vi "时间节点解密.vi"(10 "已延期":bool, 11 "输入密码":string) -> ()   [LabVIEW 2013]
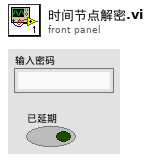
[diagram p1: front panel]
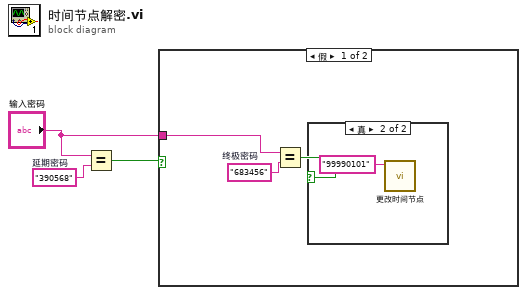
[diagram p0: block diagram]
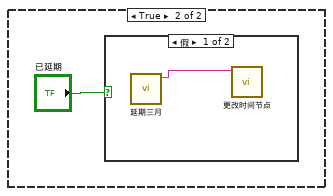
[diagram p3: hidden frame]
diagram:
  w3 = "390568"  # 延期密码
  n1 = Equal?(x="输入密码", y=w3) -> (x = y?=w2:bool)
  n2 = case shown="假" w2 {
    tunnel: "输入密码" -> [w5 _]
    frame False {
      w6 = "683456"  # 终极密码
      n3 = Equal?(x=w5, y=w6) -> (x = y?=w4:bool)
      n4 = case shown="真" w4 {
        frame False {
        }
        frame True {
          n5 = call "更改时间节点.vi"("时间字符串"="99990101") -> ()  [unwired: 10 in, 1 out]
        }
      }
    }
    frame True {
      n6 = case shown="假" "已延期" {
        frame False {
          n7 = call "延期三月.vi"() -> ("十进制整型字符串"=w9:string)  [unwired: 11 in]
          n8 = call "更改时间节点.vi"("时间字符串"=w9) -> ()  [unwired: 10 in, 1 out]
        }
        frame True {
        }
      }
    }
  }
